vi "SetPhysicalTrigger.vi"(8 "error in (no error)":errorcluster, 11 "Highland T564 DDG in":refnum<class "Highland T564 DDG.lvclass">) -> (0 "error out":errorcluster, 3 "Highland T564 DDG out":refnum<class "Highland T564 DDG.lvclass">)   [LabVIEW 2020, in "Highland T564 DDG.lvclass"]
uses:
  Highland T564 DDG.lvclass
  T560Trigger.lvclass
  C:/GEECS/Developers Version/source/Device Drivers/Highland T564 DDG/SupportLibraries/DeviceSpecific/HighlandT560Lib/T560ChannelClass/T560Channel.lvclass
  ChannelName.ctl
  Highland T564 DDG.lvclass/Highland T564 DDG.ctl
  T560Session.lvclass
  T560Channel.lvclass
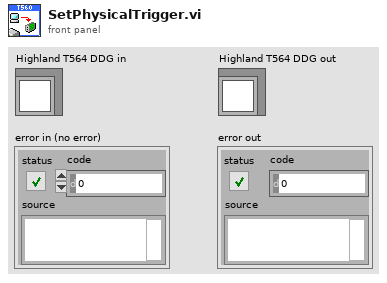
[diagram p1: front panel]
types:
  T1 = typedef "T560Channel.lvclass/ChannelName.ctl" = enum16{"Null", "A", "B", "C", "D", "Trigger"}
  T2 = typedef "Trigger.ctl" = cluster{"Divisor":T3, "Level":T3, "Impedance":T4, "Source":T5}
  T3 = typedef "Choice01.ctl" = cluster{"Value":dbl, "Min":dbl, "Max":dbl, "StepSize":dbl, "Tolerance":dbl, "ValueActual":dbl}
  T4 = typedef "TriggerImpedance.ctl" = enum16{"10KOhm", "50Ohms"}
  T5 = typedef "TriggerSource.ctl" = enum16{"Rising", "Falling", "Internal 80MHz", "Internal DDS", "Remote", "Disabled"}
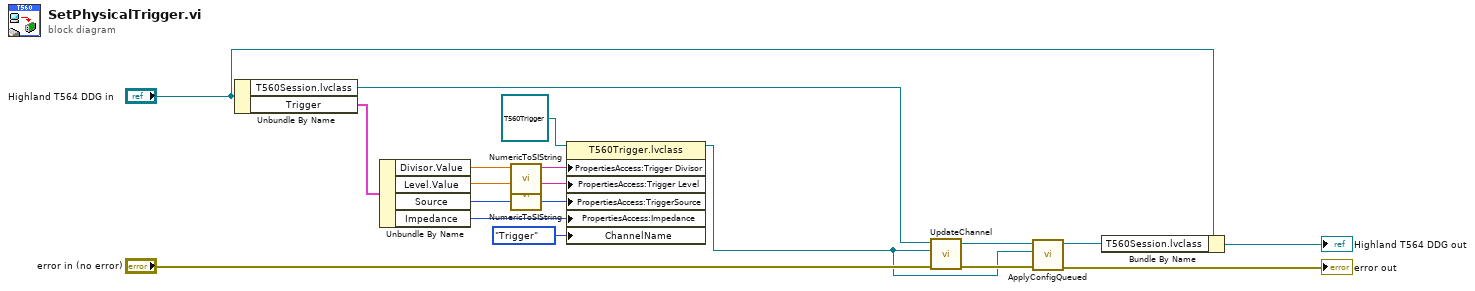
[diagram p0: block diagram]
diagram:
  n1 = Unbundle By Name("Highland T564 DDG in") -> ("T560Session.lvclass"=w4:refnum<class "T560Session.lvclass">, "Trigger"=w6:T2)
  n2 = Unbundle By Name(w6) -> ("Divisor.Value"=w7:dbl, "Level.Value"=w9:dbl, "Source"=w11:T5, "Impedance"=w3:T4)
  n3 = call "NumericToSIString.vi"("Numeric"=w7) -> ("SI_String"=w8:string)  [unwired: 9 in, 1 out]
  n4 = call "NumericToSIString.vi"("Numeric"=w9) -> ("SI_String"=w10:string)  [unwired: 9 in, 1 out]
  n5 = property class="T560Trigger.lvclass"(reference=refnum<class "T560Trigger.lvclass"> refnum ("Highlandt564.lvlib:T560Trigger.lvclass"), "PropertiesAccess:Trigger Divisor"=w8, "PropertiesAccess:Trigger Level"=w10, "PropertiesAccess:TriggerSource"=w11, "PropertiesAccess:Impedance"=w3, "ChannelName"=ChannelName."Trigger") -> (reference out=w1:refnum<class "T560Trigger.lvclass">)  [unwired: 1 in, 1 out]
  n6 = call-dynamic "UpdateChannel.vi"("error in"="error in (no error)", "UpdatedChannel.lvclass"=w1, "T560Session in"=w4) -> ("error out"=w12:errorcluster, "T560Session out"=w13:refnum<class "T560Session.lvclass">)  [unwired: 7 in]
  n7 = call-dynamic "ApplyConfigQueued.vi"("error in"=w12, "UpdatedChannel.lvclass"=w1, "T560Session in"=w13) -> ("error out"=→"error out":errorcluster, "T560Session out"=w18:refnum<class "T560Session.lvclass">)  [unwired: 7 in]
  n8 = Bundle By Name(cluster="Highland T564 DDG in", "T560Session.lvclass"=w18) -> (→"Highland T564 DDG out":refnum<class "Highland T564 DDG.lvclass">)
